vi "FTW-Actor-OnError-BeginShutdownSequence.vi"(0 "FTW Actor Instance":refnum<class "FTW-ActorInstance.lvclass">, 2 "Jobs Prior to Shutdown Sequence":string, 11 "error in":errorcluster) -> (4 "FTW Actor Instance out":refnum<class "FTW-ActorInstance.lvclass">, 15 "error out":errorcluster)   [LabVIEW 2015, in "FTW-ActorInstance.lvclass"]
uses:
  FTW-ActorInstance.lvclass
panel:
  # "Inputs"
  # "Outputs"
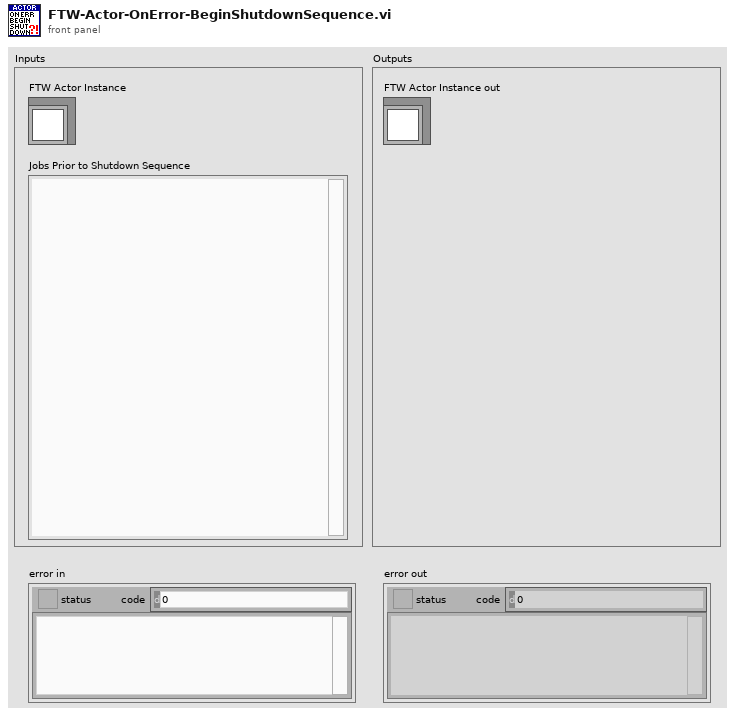
[diagram p1: front panel]
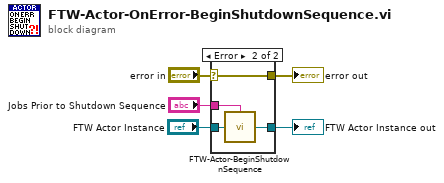
[diagram p0: block diagram]
diagram:
  n1 = case shown="Error" "error in" {
    selector: "error in" -> [w6 w8]
    tunnel: "FTW Actor Instance" -> [w7 w11]
    tunnel: [w7 w10] -> w4
    tunnel: "Jobs Prior to Shutdown Sequence" -> [_ w9]
    tunnel: [w6 w8] -> w1
    frame No Error {
    }
    frame Error {
      n2 = call "FTW-Actor-BeginShutdownSequence.vi"("Jobs Prior to Shutdown Sequence"=w9, "FTW Actor Instance"=w11) -> ("FTW Actor Instance out"=w10:refnum<class "FTW-ActorInstance.lvclass">)  [unwired: 2 in]
    }
  }
  "FTW Actor Instance out" <- w4
  "error out" <- w1
